vi "Download Waveform.vi"(0 "RFSG handle":refnum<k15>, 5 "Waveform In":T1={"Name"="Wfm", "Data"=refnum, "Signal Bandwidth (Hz)"=0.0, "PAPR (dB)"=0.0, "Burst Length (s)"=0.0, "Sample Rate"=0.0, "Burst Start Locations"=[], "Burst Stop Locations"=[], "Idle Duration Present?"=FALSE, "Runtime Scaling"=0.0, "Script"=""} {"Runtime Scaling" format="%#_6p"; "Sample Rate" format="%#_6p"; "Burst Length (s)" format="%#_6p"; "PAPR (dB)" format="%.2f"; "Signal Bandwidth (Hz)" format="%.2f"}, 11 "error in (no error)":errorcluster) -> (4 "RFSG handle out":refnum<k15>, 15 "error out":errorcluster)   [LabVIEW 2019, in "SG.lvlib"]
doc: "Downloads a previously loaded waveform to the instrument and sets associated properties."
uses:
  SG.lvlib
  Common/Waveform.ctl
  <instrlib>/niRFSG/niRFSG.llb/niRFSG Write Arb Waveform (Complex Input SGL).vi
  Common/Common.lvlib
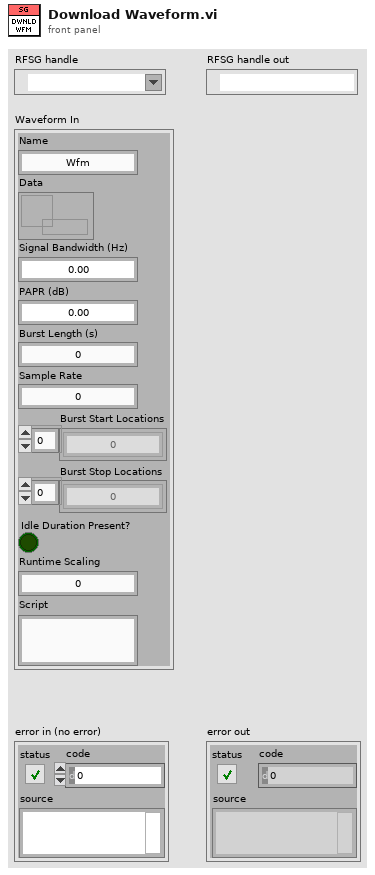
[diagram p1: front panel]
types:
  T1 = typedef "Common.lvlib/Waveform.ctl" = cluster{"Name":string, "Data":refnum<data-value>, "Signal Bandwidth (Hz)":dbl, "PAPR (dB)":dbl, "Burst Length (s)":dbl, "Sample Rate":dbl, "Burst Start Locations":i32[], "Burst Stop Locations":i32[], "Idle Duration Present?":bool, "Runtime Scaling":dbl, "Script":string}
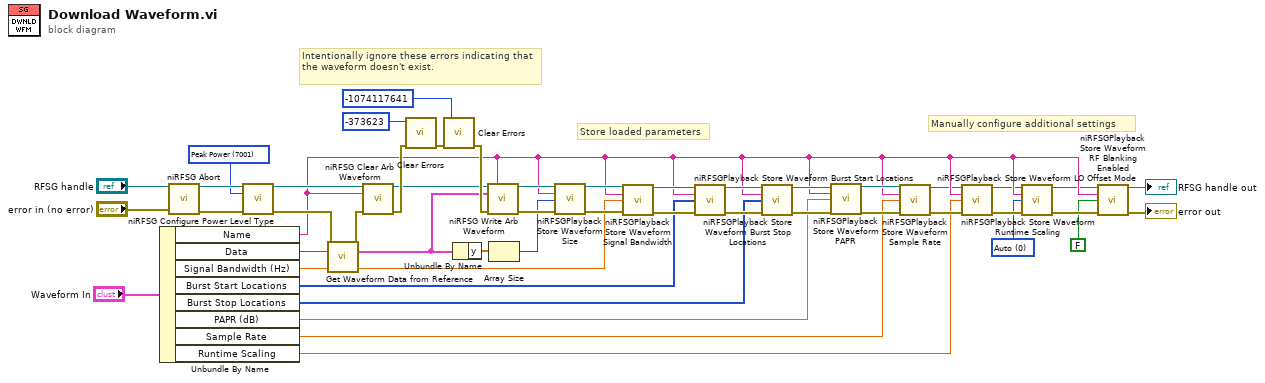
[diagram p0: block diagram]
diagram:
  w12 = 7001 items=["Average Power"=7000, "Peak Power"=7001] ("power level type")
  w28 = 0 items=["Auto", "No Offset", "Disabled"] ("LO offset mode")
  # "Manually configure additional settings"
  # "Store loaded parameters"
  # "Intentionally ignore these errors indicating that the waveform doesn't exist."
  n1 = Unbundle By Name("Waveform In") -> ("Name"=w5:string, "Data"=w8:refnum<data-value>, "Signal Bandwidth (Hz)"=w26:dbl, "Burst Start Locations"=w23:i32[], "Burst Stop Locations"=w20:i32[], "PAPR (dB)"=w19:dbl, "Sample Rate"=w15:dbl, "Runtime Scaling"=w11:dbl)
  n2 = call <instrlib>:"niRFSG Abort.vi"("instrument handle"="RFSG handle", "error in"="error in (no error)") -> ("instrument handle out"=w14:refnum<k15>, "error out"=w43:errorcluster)  [unwired: 12 in]
  n3 = call <instrlib>:"niRFSG Configure Power Level Type.vi"("instrument handle"=w14, "power level type"=w12, "error in"=w43) -> ("instrument handle out"=w13:refnum<k15>, "error out"=w33:errorcluster)  [unwired: 11 in]
  n4 = call "Get Waveform Data from Reference.vi"("Waveform Data Reference"=w8, "error in (no error)"=w33) -> ("Waveform Data"=w1:cluster{"t0":dbl, "dt":dbl, "y":csg[]}, "error out"=w32:errorcluster)  [unwired: 12 in]
  n5 = call <instrlib>:"niRFSG Clear Arb Waveform.vi"("instrument handle"=w13, "name"=w5, "error in"=w32) -> ("instrument handle out"=w27:refnum<k15>, "error out"=w42:errorcluster)  [unwired: 11 in]
  n6 = call <vilib>:"Clear Errors.vi"("error in (no error)"=w42, "specific error code to clear (0: all)"=-373623) -> ("error out"=w46:errorcluster)  [unwired: 4 in, 1 out]
  n7 = call <vilib>:"Clear Errors.vi"("error in (no error)"=w46, "specific error code to clear (0: all)"=-1074117641) -> ("error out"=w45:errorcluster)  [unwired: 4 in, 1 out]
  n8 = Unbundle By Name(w1) -> ("y"=w7:csg[])
  n9 = call-poly <instrlib>:"niRFSG Write Arb Waveform.vi"("instrument handle"=w27, "name"=w5, "IQ waveform"=w1, "error in"=w45) -> ("instrument handle out"=w10:refnum<k15>, "error out"=w38:errorcluster)  [unwired: 10 in]
  n10 = Array Size(array=w7) -> (size(s)=w6:i32)
  n11 = call <instrlib>:"niRFSGPlayback Store Waveform Size.vi"("instrument handle in"=w10, "waveform name"=w5, "waveform size"=w6, "error in"=w38) -> ("instrument handle out"=w9:refnum<k15>, "error out"=w37:errorcluster)  [unwired: 10 in]
  n12 = call <instrlib>:"niRFSGPlayback Store Waveform Signal Bandwidth.vi"("instrument handle in"=w9, "waveform name"=w5, "signal bandwidth"=w26, "error in"=w37) -> ("instrument handle out"=w24:refnum<k15>, "error out"=w44:errorcluster)  [unwired: 10 in]
  n13 = call <instrlib>:"niRFSGPlayback Store Waveform Burst Start Locations.vi"("instrument handle in"=w24, "waveform name"=w5, "burst start locations"=w23, "error in"=w44) -> ("instrument handle out"=w22:refnum<k15>, "error out"=w41:errorcluster)  [unwired: 10 in]
  n14 = call <instrlib>:"niRFSGPlayback Store Waveform Burst Stop Locations.vi"("instrument handle in"=w22, "waveform name"=w5, "burst stop locations"=w20, "error in"=w41) -> ("instrument handle out"=w21:refnum<k15>, "error out"=w40:errorcluster)  [unwired: 10 in]
  n15 = call <instrlib>:"niRFSGPlayback Store Waveform PAPR.vi"("instrument handle in"=w21, "waveform name"=w5, "PAPR"=w19, "error in"=w40) -> ("instrument handle out"=w16:refnum<k15>, "error out"=w47:errorcluster)  [unwired: 10 in]
  n16 = call <instrlib>:"niRFSGPlayback Store Waveform Sample Rate.vi"("instrument handle in"=w16, "waveform name"=w5, "sample rate"=w15, "error in"=w47) -> ("instrument handle out"=w3:refnum<k15>, "error out"=w35:errorcluster)  [unwired: 10 in]
  n17 = call <instrlib>:"niRFSGPlayback Store Waveform Runtime Scaling.vi"("instrument handle in"=w3, "waveform name"=w5, "runtime scaling"=w11, "error in"=w35) -> ("instrument handle out"=w4:refnum<k15>, "error out"=w36:errorcluster)  [unwired: 10 in]
  n18 = call <instrlib>:"niRFSGPlayback Store Waveform LO Offset Mode.vi"("instrument handle in"=w4, "waveform name"=w5, "LO offset mode"=w28, "error in"=w36) -> ("instrument handle out"=w2:refnum<k15>, "error out"=w34:errorcluster)  [unwired: 10 in]
  n19 = call <instrlib>:"niRFSGPlayback Store Waveform RF Blanking Enabled.vi"("instrument handle in"=w2, "waveform name"=w5, "RF blanking enabled"=FALSE, "error in"=w34) -> ("instrument handle out"=→"RFSG handle out":refnum<k15>, "error out"=→"error out":errorcluster)  [unwired: 10 in]
